vi "Bracket Fletcher.vi"(5 "Parsed Formula":cluster{"table":i32[][], "result":dbl[]}, 6 "loops":u32, 7 "Variables":i32[](array[numeric])=[0, 0], 8 "p":dbl[](array[numeric]) format="%.2f", 9 "xit":dbl[](array[numeric]) format="%.2f", 10 "b (start)":dbl format="%.2f", 11 "a (start)":dbl format="%.2f") -> (0 "error":i32, 1 "c (bracket)":dbl format="%.2f", 2 "b (bracket)":dbl format="%.2f", 3 "a (bracket)":dbl format="%.2f")   [LabVIEW 2010, in "NI_Gmath.lvlib"]
uses:
  NI_Gmath.lvlib
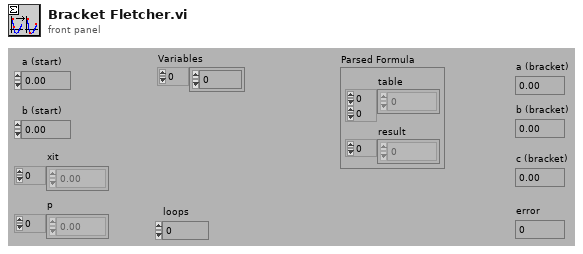
[diagram p1: front panel]
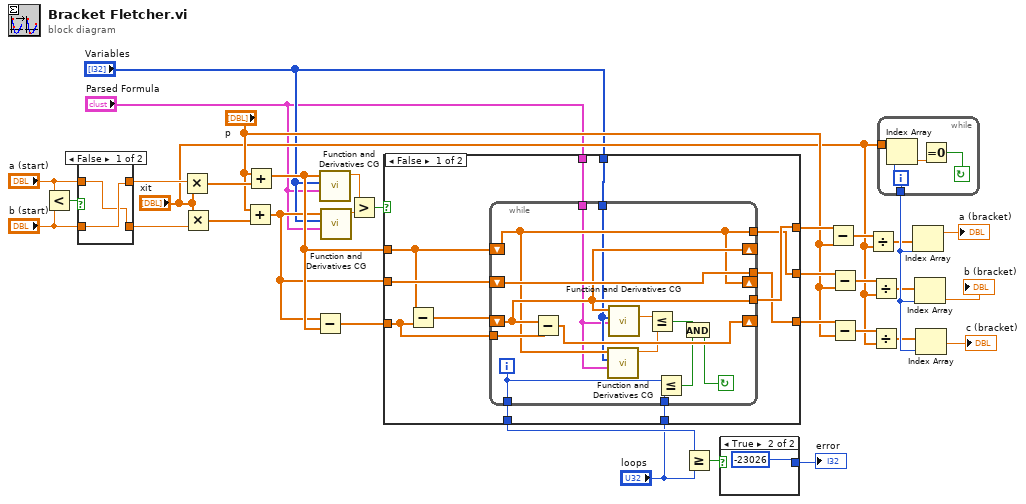
[diagram p0: block diagram]
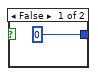
[diagram p3: hidden frame]
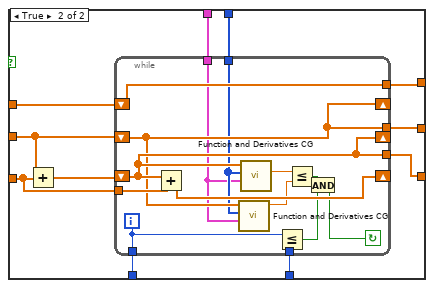
[diagram p4: hidden frame]
diagram:
  n1 = Less?(x="a (start)", y="b (start)") -> (x < y?=w28:bool)
  n2 = case shown="False" w28 {
    tunnel: "a (start)" -> [w35 w38]
    tunnel: [w36 w38] -> w24
    tunnel: "b (start)" -> [w36 w37]
    tunnel: [w35 w37] -> w21
    frame False {
    }
    frame True {
    }
  }
  n3 = Multiply(x=w24, y="xit") -> (x*y=w23:dbl[])
  n4 = Multiply(x="xit", y=w21) -> (x*y=w20:dbl[])
  n5 = Add(x="p", y=w20) -> (x+y=w19:dbl[])
  n6 = Add(x="p", y=w23) -> (x+y=w22:dbl[])
  n7 = Subtract(x=w19, y=w22) -> (x-y=w33:dbl[])
  n8 = call "Function and Derivatives CG.vi"("Parsed Formula"="Parsed Formula", "Variables"="Variables", "X"=w22) -> ("f(X)"=w3:dbl)  [unwired: 7 in, 1 out]
  n9 = call "Function and Derivatives CG.vi"("Parsed Formula"="Parsed Formula", "Variables"="Variables", "X"=w19) -> ("f(X)"=w26:dbl)  [unwired: 7 in, 1 out]
  n10 = Greater?(x=w3, y=w26) -> (0:w34:bool)
  n11 = case shown="False" w34 {
    tunnel: w22 -> [w46 w74]
    tunnel: w19 -> [w47 w73]
    tunnel: w33 -> [w44 w71]
    tunnel: [w43 w68] -> w18
    tunnel: [w42 w67] -> w16
    tunnel: [w41 w66] -> w15
    tunnel: [w49 w70] -> w32
    tunnel: "loops" -> [w48 w69]
    tunnel: "Variables" -> [w40 w65]
    tunnel: "Parsed Formula" -> [w39 w64]
    frame False {
      n12 = Subtract(x=w46, y=w44) -> (x-y=w45:dbl[])
      n13 = while {
        tunnel: [w55] -> w41
        tunnel: [w53] -> w42
        tunnel: [w54] -> w43
        tunnel: w48 -> [w59]
        tunnel: [w60] -> w49
        tunnel: w44 -> [w63]
        shift-left: w45 -> [w54]
        shift-right: [w61] -> _
        shift-left: w47 -> [w55]
        shift-right: [w53] -> _
        shift-left: w46 -> [w53]
        shift-right: [w54] -> _
        tunnel: w40 -> [w51]
        tunnel: w39 -> [w50]
        i -> [w60]
        stop <- w56 continue-if-true
        n14 = Subtract(x=w54, y=w63) -> (x-y=w61:dbl[])
        n15 = call "Function and Derivatives CG.vi"("Parsed Formula"=w50, "Variables"=w51, "X"=w53) -> ("f(X)"=w52:dbl)  [unwired: 7 in, 1 out]
        n16 = call "Function and Derivatives CG.vi"("Parsed Formula"=w50, "Variables"=w51, "X"=w54) -> ("f(X)"=w62:dbl)  [unwired: 7 in, 1 out]
        n17 = Less Or Equal?(x=w62, y=w52) -> (x <= y?=w58:bool)
        n18 = Less Or Equal?(x=w60, y=w59) -> (x <= y?=w57:bool)
        n19 = And(x=w58, y=w57) -> (x .and. y?=w56:bool)
      }
    }
    frame True {
      n20 = Add(x=w73, y=w71) -> (x+y=w72:dbl[])
      n21 = while {
        tunnel: [w79] -> w66
        tunnel: [w78] -> w67
        tunnel: [w80] -> w68
        tunnel: w69 -> [w84]
        tunnel: [w85] -> w70
        tunnel: w71 -> [w88]
        shift-left: w72 -> [w79]
        shift-right: [w86] -> _
        shift-left: w73 -> [w78]
        shift-right: [w79] -> _
        shift-left: w74 -> [w80]
        shift-right: [w78] -> _
        tunnel: w65 -> [w76]
        tunnel: w64 -> [w75]
        i -> [w85]
        stop <- w81 continue-if-true
        n22 = Add(x=w79, y=w88) -> (x+y=w86:dbl[])
        n23 = call "Function and Derivatives CG.vi"("Parsed Formula"=w75, "Variables"=w76, "X"=w78) -> ("f(X)"=w77:dbl)  [unwired: 7 in, 1 out]
        n24 = call "Function and Derivatives CG.vi"("Parsed Formula"=w75, "Variables"=w76, "X"=w79) -> ("f(X)"=w87:dbl)  [unwired: 7 in, 1 out]
        n25 = Less Or Equal?(x=w85, y=w84) -> (x <= y?=w82:bool)
        n26 = Less Or Equal?(x=w87, y=w77) -> (x <= y?=w83:bool)
        n27 = And(x=w83, y=w82) -> (x .and. y?=w81:bool)
      }
    }
  }
  n28 = Greater Or Equal?(x=w32, y="loops") -> (x >= y?=w30:bool)
  n29 = case shown="True" w30 {
    tunnel: [0 -23026] -> w29
    frame False {
    }
    frame True {
    }
  }
  "error" <- w29
  n30 = Subtract(x=w18, y="p") -> (x-y=w17:dbl[])
  n31 = Subtract(x=w16, y="p") -> (x-y=w13:dbl[])
  n32 = Subtract(x=w15, y="p") -> (x-y=w12:dbl[])
  n33 = Divide(x=w17, y="xit") -> (x/y=w9:dbl[])
  n34 = Divide(x=w13, y="xit") -> (x/y=w8:dbl[])
  n35 = Divide(x=w12, y="xit") -> (x/y=w7:dbl[])
  n36 = while {
    tunnel: [w93] -> w10
    tunnel: "xit" -> [w94]
    i -> [w93]
    stop <- w91 continue-if-true
    n37 = Index Array(array=w94, index=w93) -> (element=w92:dbl)
    n38 = Equal To 0?(x=w92) -> (x = 0?=w91:bool)
  }
  n39 = Index Array(array=w9, index=w10) -> (element=→"a (bracket)":dbl)
  n40 = Index Array(array=w8, index=w10) -> (element=→"b (bracket)":dbl)
  n41 = Index Array(array=w7, index=w10) -> (element=→"c (bracket)":dbl)
